vi "SCCSup Dialog_GenMCLB_Filter.vi"(6 "current selection":string, 9 "filter column":i32, 10 "filter string":string, 11 "complete item names":string[][](array[string])) -> (1 "filter string row index":i32, 3 "filtered item names":string[][](array[string]))   [LabVIEW 2017]
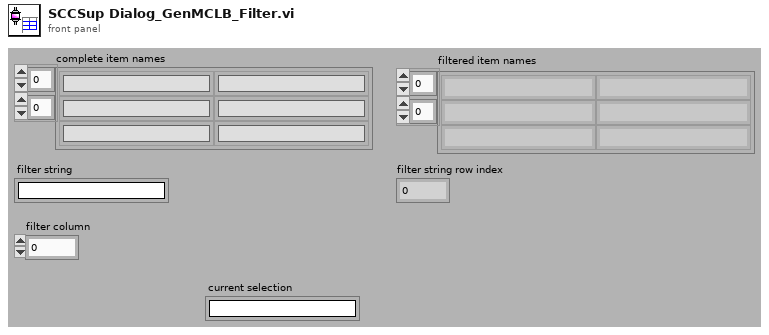
[diagram p1: front panel]
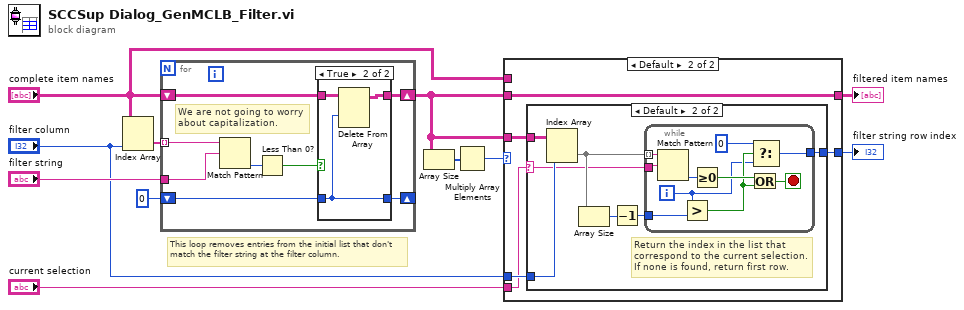
[diagram p0: block diagram]
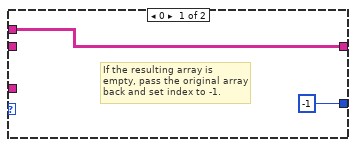
[diagram p2: hidden frame]
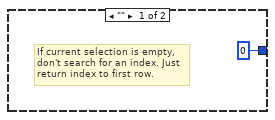
[diagram p3: hidden frame]
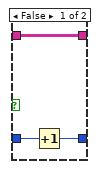
[diagram p4: hidden frame]
diagram:
  # "This loop removes entries from the initial list that don't match the filter string at the filter column."
  n1 = Index Array(array="complete item names", index (col)="filter column") -> (element=w10:string[])  [unwired: 1 in]
  n2 = for {
    tunnel: w10 -> [w12] mode=indexing
    tunnel: "filter string" -> [w19]
    shift-right: [w14] -> _
    shift-left: 0 ("index") -> [w15]
    shift-right: [w13] -> w6
    shift-left: "complete item names" -> [w16]
    # "We are not going to worry about capitalization."
    n3 = Match Pattern(string=w12, regular expression=w19) -> (offset past match=w17:i32)  [unwired: 1 in, 3 out]
    n4 = Less Than 0?(x=w17) -> (x < 0?=w18:bool)
    n5 = case shown="True" w18 {
      tunnel: w16 -> [w20 w25]
      tunnel: w15 -> [w22 w24]
      tunnel: [w21 w24] -> w14
      tunnel: [w20 w23] -> w13
      frame False {
        n6 = Increment(x=w22) -> (x+1=w21:i32)
      }
      frame True {
        n7 = Delete From Array(array=w25, index (row)=w24) -> (array with subset deleted=w23:string[][])  [unwired: 2 in, 1 out]
      }
    }
  }
  n8 = Array Size(array=w6) -> (size(s)=w7:i32[])
  n9 = Multiply Array Elements(1:w7) -> (0:w1:i32)
  n10 = case shown="Default" w1 {
    tunnel: "filter column" -> [_ w32]
    tunnel: "current selection" -> [_ w28]
    tunnel: [-1 ("t") w31] -> w8
    tunnel: w6 -> [_ w30]
    tunnel: w6 -> [_ w29]
    tunnel: [w26 w29] -> w5
    tunnel: "complete item names" -> [w26 _]
    frame 0 {
      # "If the resulting array is empty, pass the original array back and set index to -1."
    }
    frame Default {
      n11 = case shown="Default" w28 {
        selector: w28 -> [_ w34]
        tunnel: w32 -> [_ w40]
        tunnel: [0 ("t") w36] -> w31
        tunnel: w30 -> [_ w35]
        frame "" {
          # "If current selection is empty, don't search for an index. Just return index to first row."
        }
        frame Default {
          # "Return the index in the list that correspond to the current selection. If none is found, return first row."
          n12 = Index Array(array=w35, index (col)=w40) -> (element=w38:string[])  [unwired: 1 in]
          n13 = Array Size(array=w38) -> (size(s)=w39:i32)
          n14 = Decrement(x=w39) -> (x-1=w37:i32)
          n15 = while {
            tunnel: w38 -> [w43] mode=indexing
            tunnel: w34 -> [w42]
            tunnel: w37 -> [w49]
            tunnel: [w45] -> w36
            i -> [w41]
            stop <- w48 stop-if-true
            n16 = Match Pattern(string=w43, regular expression=w42) -> (offset past match=w44:i32)  [unwired: 1 in, 3 out]
            n17 = Greater?(x=w41, y=w49) -> (0:w47:bool)
            n18 = Greater Or Equal To 0?(x=w44) -> (x >= 0?=w50:bool)
            n19 = Or(x=w50, y=w47) -> (x .or. y?=w48:bool)
            n20 = Select(t=0, s=w47, f=w41) -> (s? t:f=w45:i32)
          }
        }
      }
    }
  }
  "filtered item names" <- w5
  "filter string row index" <- w8
